vi "Write XNET Frame.vi"(8 "error in (no error)":errorcluster, 10 "XNET Frame":refnum<k21>, 11 "XNET Data in":refnum<class "XNET Data.lvclass">) -> (0 "error out":errorcluster, 3 "XNET Data out":refnum<class "XNET Data.lvclass">)   [LabVIEW 2021, in "BS120x Driver.lvlib" / "Data Classes.lvlib" / "XNET Data.lvclass"]
uses:
  XNET Data.lvclass
  XNET Data.lvclass/XNET Data.ctl
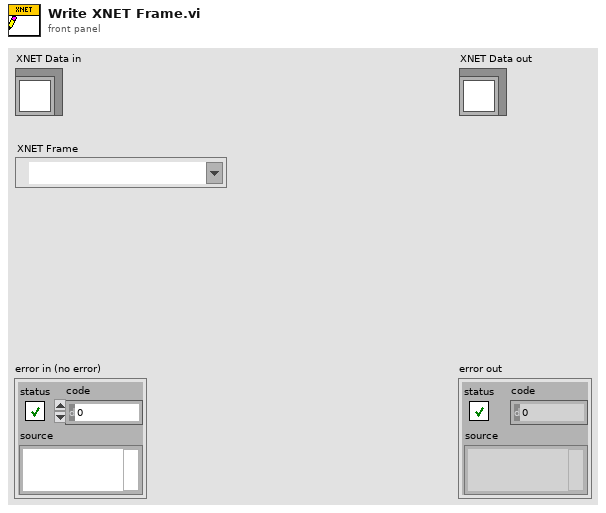
[diagram p1: front panel]
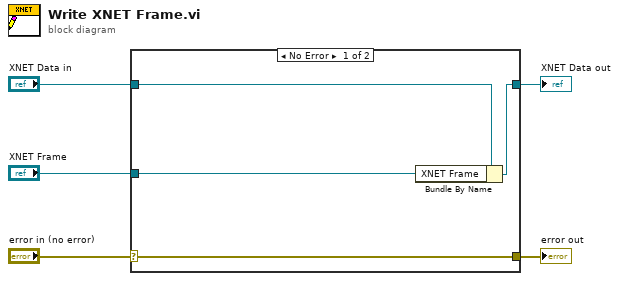
[diagram p0: block diagram]
diagram:
  n1 = case shown="No Error" "error in (no error)" {
    selector: "error in (no error)" -> [w9 w10]
    tunnel: [w9 w10] -> w4
    tunnel: [w7 w11] -> w2
    tunnel: "XNET Data in" -> [w8 w11]
    tunnel: "XNET Frame" -> [w6 _]
    frame No Error {
      n2 = Bundle By Name(cluster=w8, "XNET Frame"=w6) -> (w7:refnum<class "XNET Data.lvclass">)
    }
    frame Error {
    }
  }
  "error out" <- w4
  "XNET Data out" <- w2
